vi "VISA Write .vi"() -> ()   [LabVIEW 2016]
uses:
  <vilib>/Instr/_visa.llb/VISA Configure Serial Port (Instr).vi
panel:
  out "return count 3":u32
  out "return count 2":u32
  out "return count":u32
  in  "VISA resource name 3":refnum<visa-resource-name>
  in  "VISA resource name 2":refnum<visa-resource-name>
  in  "VISA resource name":refnum<visa-resource-name>
  in  "green":bool
  in  "red":bool
  in  "blue":bool
  in  "STOP":bool
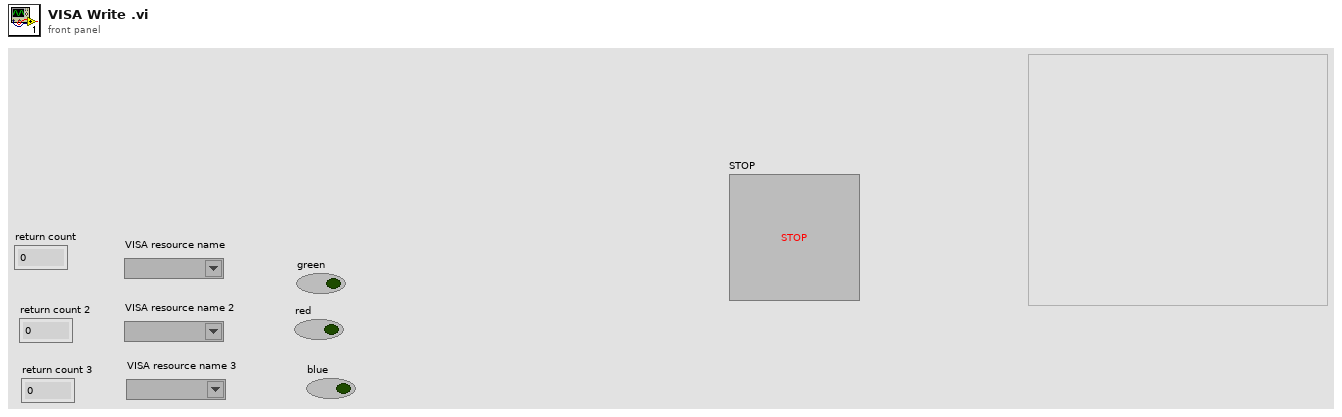
[diagram p1: front panel]
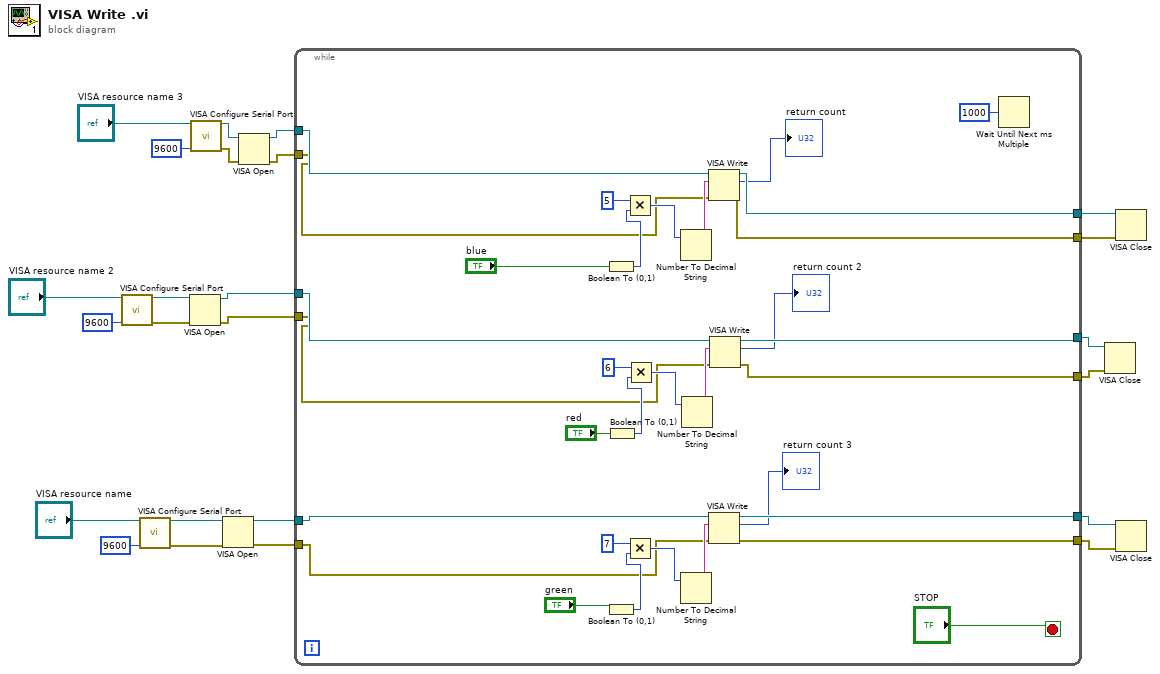
[diagram p0: block diagram]
diagram:
  n1 = call-poly "VISA Configure Serial Port"("VISA resource name"="VISA resource name 2", "baud rate (9600)"=u32 9600) -> ("VISA resource name out"=w16:refnum<visa-resource-name>, "error out"=w13:errorcluster)  [unwired: 12 in]
  n2 = call-poly "VISA Configure Serial Port"("VISA resource name"="VISA resource name", "baud rate (9600)"=u32 9600) -> ("VISA resource name out"=w9:refnum<visa-resource-name>, "error out"=w8:errorcluster)  [unwired: 12 in]
  n3 = VISA Open(error in (no error)=w13, VISA resource name=w16) -> (VISA resource name=w15:refnum<visa-resource-name>, error out=w14:errorcluster)  [unwired: 3 in]
  n4 = call-poly "VISA Configure Serial Port"("VISA resource name"="VISA resource name 3", "baud rate (9600)"=u32 9600) -> ("VISA resource name out"=w23:refnum<visa-resource-name>, "error out"=w24:errorcluster)  [unwired: 12 in]
  n5 = VISA Open(error in (no error)=w8, VISA resource name=w9) -> (VISA resource name=w7:refnum<visa-resource-name>, error out=w6:errorcluster)  [unwired: 3 in]
  n6 = VISA Open(error in (no error)=w24, VISA resource name=w23) -> (VISA resource name=w22:refnum<visa-resource-name>, error out=w21:errorcluster)  [unwired: 3 in]
  n7 = while {
    tunnel: w22 -> [w47]
    tunnel: w21 -> [w46]
    tunnel: [w45] -> w20
    tunnel: [w44] -> w19
    tunnel: [w43] -> w18
    tunnel: [w42] -> w17
    tunnel: w15 -> [w49]
    tunnel: w14 -> [w48]
    tunnel: w7 -> [w35]
    tunnel: w6 -> [w34]
    tunnel: [w33] -> w5
    tunnel: [w32] -> w4
    stop <- "STOP" stop-if-true
    n8 = Boolean To (0,1)(Boolean="blue") -> (0, 1=w54:i16)
    n9 = Boolean To (0,1)(Boolean="green") -> (0, 1=w38:i16)
    n10 = Boolean To (0,1)(Boolean="red") -> (0, 1=w51:i16)
    n11 = Multiply(x=i16 5, y=w54) -> (x*y=w55:i16)
    n12 = Multiply(x=i16 7, y=w38) -> (x*y=w39:i16)
    n13 = Multiply(x=i16 6, y=w51) -> (x*y=w52:i16)
    n14 = Number To Decimal String(number=w55) -> (decimal integer string=w53:string)  [unwired: 1 in]
    n15 = Number To Decimal String(number=w39) -> (decimal integer string=w37:string)  [unwired: 1 in]
    n16 = Number To Decimal String(number=w52) -> (decimal integer string=w50:string)  [unwired: 1 in]
    n17 = VISA Write(VISA resource name=w47, write buffer=w53, error in (no error)=w46) -> (VISA resource name out=w45:refnum<visa-resource-name>, return count=→"return count":u32, error out=w44:errorcluster)
    n18 = VISA Write(VISA resource name=w35, write buffer=w37, error in (no error)=w34) -> (VISA resource name out=w33:refnum<visa-resource-name>, return count=→"return count 3":u32, error out=w32:errorcluster)
    n19 = VISA Write(VISA resource name=w49, write buffer=w50, error in (no error)=w48) -> (VISA resource name out=w43:refnum<visa-resource-name>, return count=→"return count 2":u32, error out=w42:errorcluster)
    n20 = Wait Until Next ms Multiple(millisecond multiple=u32 1000) -> ()  [unwired: 1 out]
  }
  n21 = VISA Close(VISA resource name=w18, error in (no error)=w17) -> ()  [unwired: 1 out]
  n22 = VISA Close(VISA resource name=w20, error in (no error)=w19) -> ()  [unwired: 1 out]
  n23 = VISA Close(VISA resource name=w5, error in (no error)=w4) -> ()  [unwired: 1 out]
